vi "Function_Generator2.vi"() -> ()   [LabVIEW 2013]
uses:
  <vilib>/express/express analysis/Spectral/Block/exnSpectralBlock spectral measurements peak poly.vi
  <vilib>/express/express analysis/Spectral/Block/exnSpectralBlock spectral measurements peak DDT.vi
  <vilib>/express/express analysis/Spectral/XNode/ExpressSpectralMeasurementsBlockNode.xnode
panel:
  out ".not. x?":bool
  in  "File save selector":T1(radio)
  out "Recorded time":dbl
  in  "Record & Stop Button":bool
  in  "Radio Buttons":T1(radio)
  in  "Jpg imgae button":bool
  in  "Tab Control":enum32{"Waveform", "FFT"}(tab)
  out "Waveform Graph 2":dynamicdata(graph) caption="Waveform Graph"
  out "FFT":dynamicdata(graph)
  in  "Noise on/off":bool
  in  "ms/Div":i32(knob) scale=0.0..4.0 scale format="%.0g"
  in  "Volt/Div":dbl(knob) scale=0.0..4.0 scale format="%_2g"
  in  "Offset":i32(slide) scale=-5.0..5.0
  in  "Frequency":dbl(knob) scale=10.0..20.0 scale format="%#_2p"
  in  "Freq mutiplier":dbl(slide) caption="Multiplier" scale=2.0..1000.0
  in  "Trigger":bool
  out "DC":bool
  out "Square":bool
  out "Sawtooth":bool
  out "Traingle":bool
  out "Sine":bool
  out "Frequency":dbl format="%#_3pHz"
  out "Peak to Peak Amplitude":dbl format="%#_3gV"
  in  "Noise":i32(knob) scale=0.0..2.0
  in  "Phase":dbl(knob) scale=0.0..360.0 scale format="%.0p"
  in  "Signal type":i32(knob) step=1 scale=0.0..4.0
  in  "Amplitude":dbl(knob) scale=0.0..10.0
  in  "stop":bool
  in  "Duty Cycle (%)":dbl(knob)=50.0 scale=0.0..100.0
  in  "Standered deviation":dbl(slide) scale=-1.0..1.0 scale format="%#_1g"
  in  "Noise Amplitude":dbl(slide) scale=0.0..5.0
  in  "FFT save button":bool
  in  "Trail probability":dbl(slide) scale=0.0..1.0 scale format="%#.1g"
  # "Function Generator / Oscilloscope"
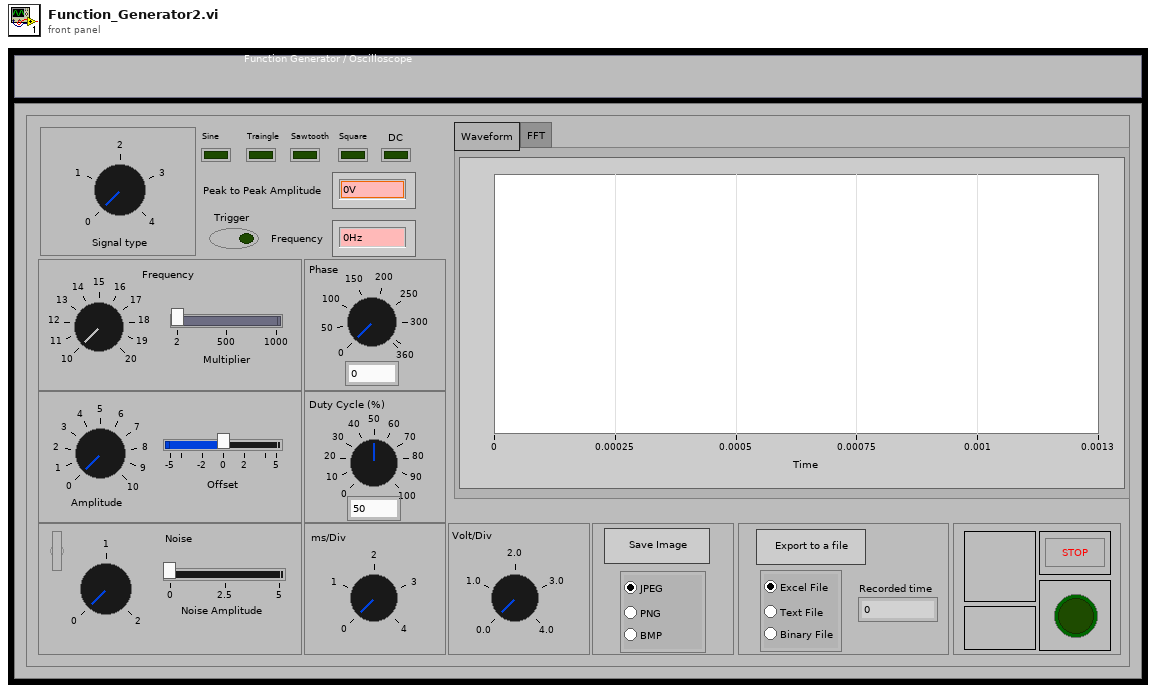
[diagram p1: front panel]
types:
  T1 = enum32{"Radio Selection 1", "Radio Selection 2", "Radio Selection 3"}
  T2 = cluster{"averaging mode":u16, "weighting mode":u16, "number of averages":u32}
  T3 = cluster{"dB On (F)":bool, "unwrap phase (F)":bool, "convert to degree (F)":bool}
  T4 = typedef "imagedata.ctl" = cluster{"image type":i32, "image depth":i32, "image":u8[], "mask":u8[], "colors":u32[], "Rectangle":cluster{"left":i16, "top":i16, "right":i16, "bottom":i16}}
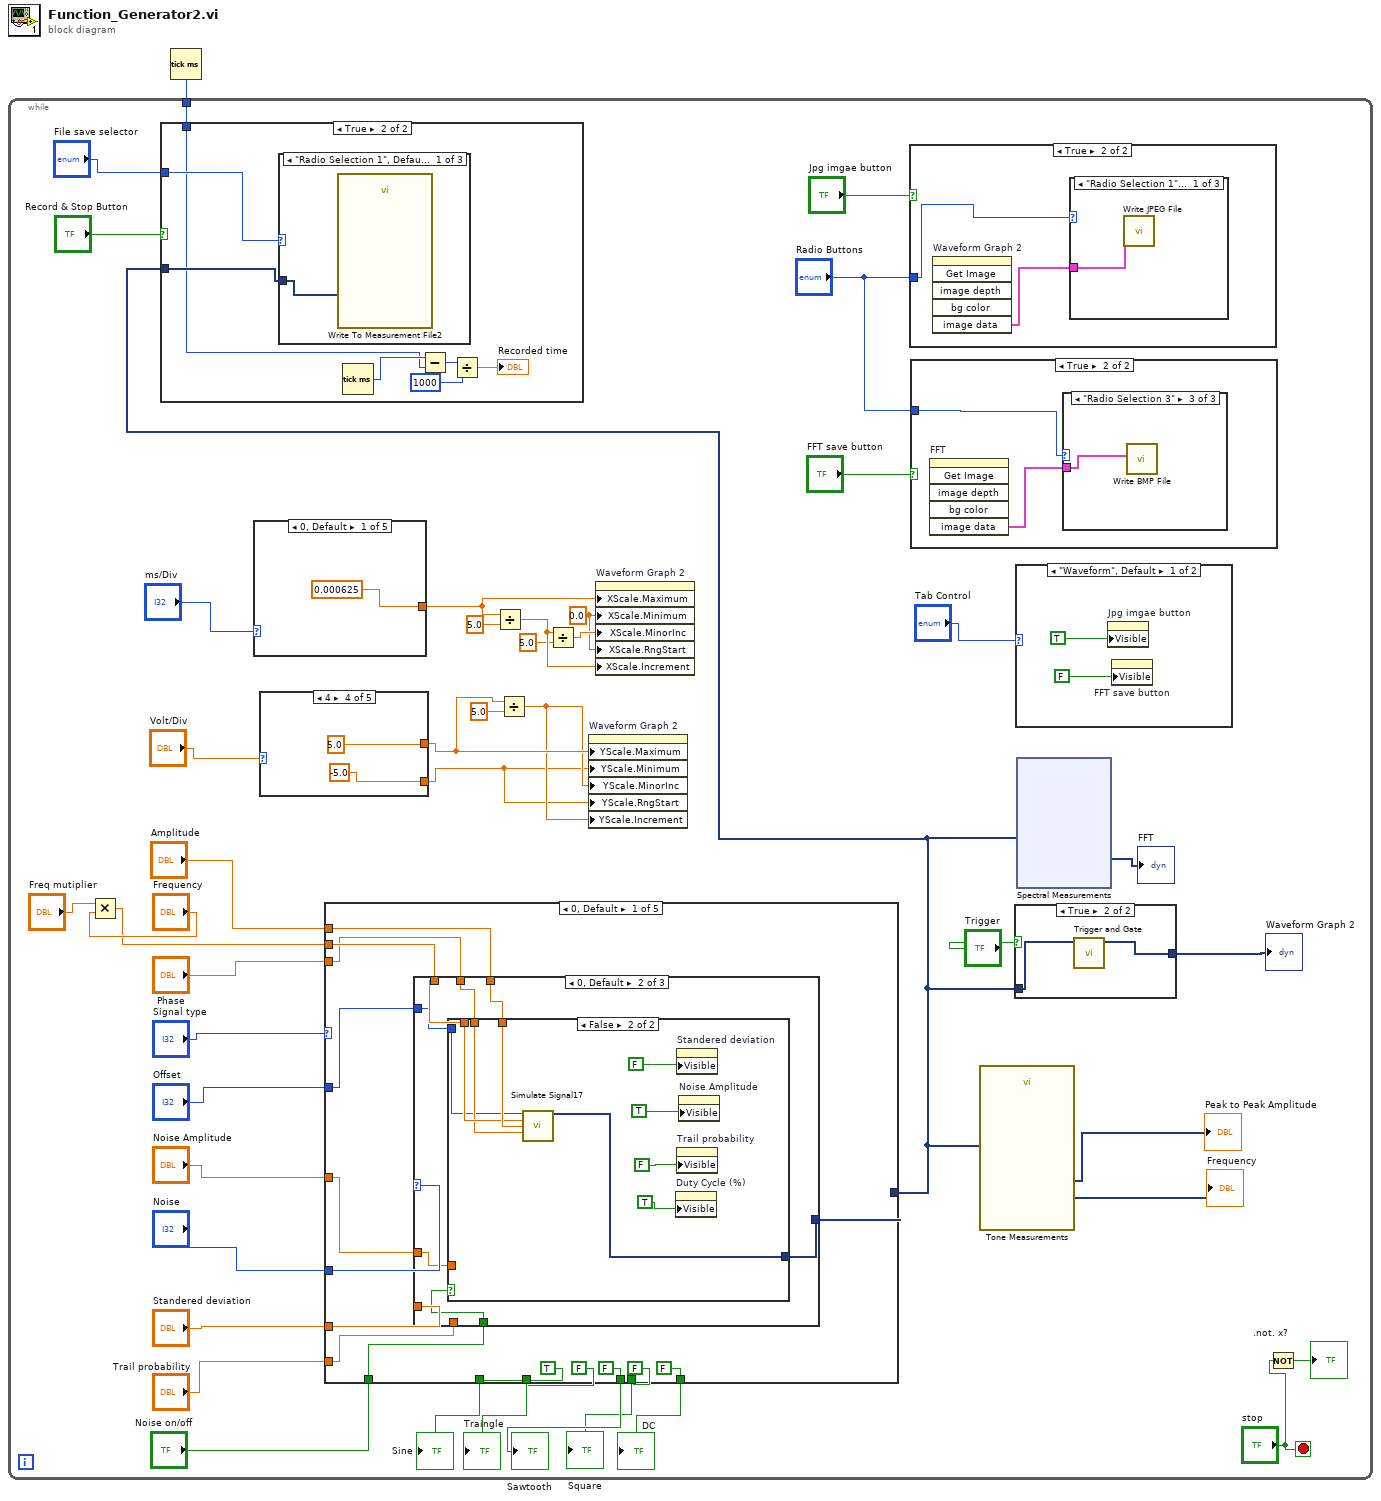
[diagram p0: block diagram]
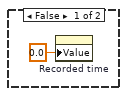
[diagram p2: hidden frame]
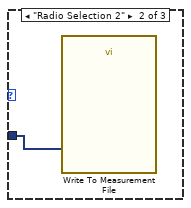
[diagram p3: hidden frame]
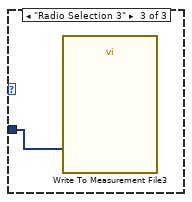
[diagram p4: hidden frame]
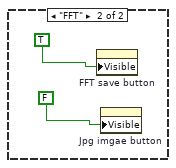
[diagram p5: hidden frame]
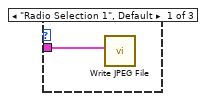
[diagram p7: hidden frame]
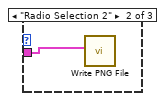
[diagram p8: hidden frame]
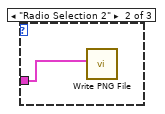
[diagram p10: hidden frame]
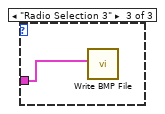
[diagram p11: hidden frame]
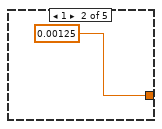
[diagram p12: hidden frame]
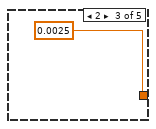
[diagram p13: hidden frame]
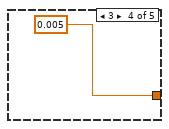
[diagram p14: hidden frame]
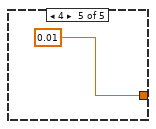
[diagram p15: hidden frame]
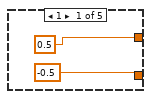
[diagram p16: hidden frame]
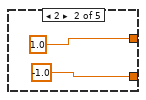
[diagram p17: hidden frame]
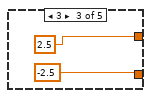
[diagram p18: hidden frame]
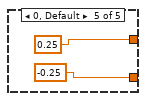
[diagram p19: hidden frame]
diagram:
  n1 = Tick Count (ms)() -> (millisecond timer value=w1:u32)
  n2 = while {
    tunnel: w1 -> [w6]
    stop <- "stop" stop-if-true
    w14 = 0.0 ("X Scale.Range:Minimum")
    n3 = Multiply(x="Freq mutiplier", y="Frequency") -> (x*y=w27:dbl)
    n4 = case shown="0, Default" "ms/Div" {
      tunnel: [0.000625 0.00125 0.0025 0.005 0.01] -> w19
      frame 0, Default {
      }
      frame 1 {
      }
      frame 2 {
      }
      frame 3 {
      }
      frame 4 {
      }
    }
    n5 = case shown="4" "Volt/Div" {
      tunnel: [0.5 1.0 2.5 5.0 0.25] -> w23
      tunnel: [-0.5 -1.0 -2.5 -5.0 -0.25] -> w21
      frame 1 {
      }
      frame 2 {
      }
      frame 3 {
      }
      frame 4 {
      }
      frame 0, Default {
      }
    }
    n6 = case shown="0, Default" "Signal type" {
      tunnel: "Amplitude" -> [w113 w204 w298 w389 _]
      tunnel: w27 -> [w112 w203 w297 w388 _]
      tunnel: "Phase" -> [w111 w202 w296 w387 _]
      tunnel: "Offset" -> [w110 w199 w295 w386 w488]
      tunnel: "Noise Amplitude" -> [w108 w205 w294 w385 w487]
      tunnel: "Noise" -> [w105 w206 w299 w390 w489]
      tunnel: "Standered deviation" -> [w109 w200 w292 w383 w485]
      tunnel: "Trail probability" -> [w107 w198 w291 w382 w484]
      tunnel: [w106 w201 w293 w384 w486] -> w7
      tunnel: [TRUE FALSE FALSE FALSE FALSE] -> w36
      tunnel: [FALSE TRUE FALSE FALSE FALSE] -> w35
      tunnel: [FALSE FALSE TRUE FALSE FALSE] -> w34
      tunnel: [FALSE FALSE FALSE TRUE FALSE] -> w33
      tunnel: [FALSE FALSE FALSE FALSE TRUE] -> w32
      tunnel: "Noise on/off" -> [w99 w192 w285 w375 w478]
      frame 0, Default {
        n7 = case shown="0, Default" w105 {
          tunnel: w113 -> [w120 w146 w172]
          tunnel: w112 -> [w118 w145 w171]
          tunnel: w111 -> [w119 w144 w170]
          tunnel: w110 -> [w115 w143 w169]
          tunnel: w109 -> [_ _ w168]
          tunnel: w108 -> [_ w142 _]
          tunnel: w107 -> [w117 _ _]
          tunnel: [w116 w141 w167] -> w106
          tunnel: w99 -> [w114 w140 w166]
          frame 2 {
            n8 = case shown="False" w114 {
              tunnel: w120 -> [w130 w139]
              tunnel: w119 -> [w129 w138]
              tunnel: w118 -> [w128 w137]
              tunnel: w117 -> [w127 _]
              tunnel: [w123 w133] -> w116
              tunnel: w115 -> [w121 w131]
              frame True {
                n9 = call "Simulate Signal3"("Offset"=w121, "Frequency"=w128, "Amplitude"=w130, "Phase"=w129, "Trial probability"=w127) -> ("Sine with Binomial Noise"=w123:dynamicdata)  [unwired: 9 in, 1 out]
                n10 = property on="Duty Cycle (%)" class="Knob (strict)"("Visible"=TRUE) -> ()  [unwired: 2 in, 2 out]
                n11 = property on="Noise Amplitude" class="Slide (strict)"("Visible"=FALSE) -> ()  [unwired: 2 in, 2 out]
                n12 = property on="Trail probability" class="Slide (strict)"("Visible"=TRUE) -> ()  [unwired: 2 in, 2 out]
                n13 = property on="Standered deviation" class="Slide (strict)"("Visible"=FALSE) -> ()  [unwired: 2 in, 2 out]
              }
              frame False {
                n14 = call "Simulate Signal18"("Offset"=w131, "Frequency"=w137, "Amplitude"=w139, "Phase"=w138) -> ("Sine"=w133:dynamicdata)  [unwired: 10 in, 1 out]
                n15 = property on="Duty Cycle (%)" class="Knob (strict)"("Visible"=TRUE) -> ()  [unwired: 2 in, 2 out]
                n16 = property on="Noise Amplitude" class="Slide (strict)"("Visible"=FALSE) -> ()  [unwired: 2 in, 2 out]
                n17 = property on="Trail probability" class="Slide (strict)"("Visible"=TRUE) -> ()  [unwired: 2 in, 2 out]
                n18 = property on="Standered deviation" class="Slide (strict)"("Visible"=FALSE) -> ()  [unwired: 2 in, 2 out]
              }
            }
          }
          frame 0, Default {
            n19 = case shown="False" w140 {
              tunnel: w146 -> [w156 w165]
              tunnel: w145 -> [w155 w164]
              tunnel: w144 -> [w154 w163]
              tunnel: w143 -> [w153 w162]
              tunnel: w142 -> [w152 _]
              tunnel: [w148 w158] -> w141
              frame True {
                n20 = call "Simulate Signal"("Offset"=w153, "Frequency"=w155, "Amplitude"=w156, "Phase"=w154, "Noise amplitude"=w152) -> ("Sine with Uniform Noise"=w148:dynamicdata)  [unwired: 9 in, 1 out]
                n21 = property on="Duty Cycle (%)" class="Knob (strict)"("Visible"=TRUE) -> ()  [unwired: 2 in, 2 out]
                n22 = property on="Standered deviation" class="Slide (strict)"("Visible"=FALSE) -> ()  [unwired: 2 in, 2 out]
                n23 = property on="Trail probability" class="Slide (strict)"("Visible"=FALSE) -> ()  [unwired: 2 in, 2 out]
                n24 = property on="Noise Amplitude" class="Slide (strict)"("Visible"=TRUE) -> ()  [unwired: 2 in, 2 out]
              }
              frame False {
                n25 = call "Simulate Signal17"("Offset"=w162, "Frequency"=w164, "Amplitude"=w165, "Phase"=w163) -> ("Sine"=w158:dynamicdata)  [unwired: 10 in, 1 out]
                n26 = property on="Duty Cycle (%)" class="Knob (strict)"("Visible"=TRUE) -> ()  [unwired: 2 in, 2 out]
                n27 = property on="Standered deviation" class="Slide (strict)"("Visible"=FALSE) -> ()  [unwired: 2 in, 2 out]
                n28 = property on="Trail probability" class="Slide (strict)"("Visible"=FALSE) -> ()  [unwired: 2 in, 2 out]
                n29 = property on="Noise Amplitude" class="Slide (strict)"("Visible"=TRUE) -> ()  [unwired: 2 in, 2 out]
              }
            }
          }
          frame 1 {
            n30 = case shown="True" w166 {
              tunnel: w172 -> [w182 w191]
              tunnel: w171 -> [w181 w190]
              tunnel: w170 -> [w180 w189]
              tunnel: w169 -> [w179 w188]
              tunnel: w168 -> [w178 _]
              tunnel: [w174 w184] -> w167
              frame True {
                n31 = call "Simulate Signal2"("Offset"=w179, "Frequency"=w181, "Amplitude"=w182, "Phase"=w180, "Standard deviation"=w178) -> ("Sine with Gaussian Noise"=w174:dynamicdata)  [unwired: 9 in, 1 out]
                n32 = property on="Noise Amplitude" class="Slide (strict)"("Visible"=FALSE) -> ()  [unwired: 2 in, 2 out]
                n33 = property on="Standered deviation" class="Slide (strict)"("Visible"=TRUE) -> ()  [unwired: 2 in, 2 out]
                n34 = property on="Trail probability" class="Slide (strict)"("Visible"=FALSE) -> ()  [unwired: 2 in, 2 out]
                n35 = property on="Duty Cycle (%)" class="Knob (strict)"("Visible"=TRUE) -> ()  [unwired: 2 in, 2 out]
              }
              frame False {
                n36 = call "Simulate Signal16"("Offset"=w188, "Frequency"=w190, "Amplitude"=w191, "Phase"=w189) -> ("Sine"=w184:dynamicdata)  [unwired: 10 in, 1 out]
                n37 = property on="Noise Amplitude" class="Slide (strict)"("Visible"=FALSE) -> ()  [unwired: 2 in, 2 out]
                n38 = property on="Standered deviation" class="Slide (strict)"("Visible"=TRUE) -> ()  [unwired: 2 in, 2 out]
                n39 = property on="Trail probability" class="Slide (strict)"("Visible"=FALSE) -> ()  [unwired: 2 in, 2 out]
                n40 = property on="Duty Cycle (%)" class="Knob (strict)"("Visible"=TRUE) -> ()  [unwired: 2 in, 2 out]
              }
            }
          }
        }
      }
      frame 1 {
        n41 = case shown="1" w206 {
          tunnel: w205 -> [w213 _ w261]
          tunnel: w204 -> [w212 w238 w264]
          tunnel: w203 -> [w211 w237 w263]
          tunnel: w202 -> [w210 w236 w262]
          tunnel: [w209 w234 w260] -> w201
          tunnel: w200 -> [_ w239 _]
          tunnel: w199 -> [w208 w235 _]
          tunnel: w198 -> [_ _ w265]
          tunnel: w192 -> [w207 w233 w259]
          frame 0, Default {
            n42 = case shown="False" w207 {
              tunnel: w213 -> [w223 _]
              tunnel: w212 -> [w222 w232]
              tunnel: w211 -> [w221 w231]
              tunnel: w210 -> [w220 w230]
              tunnel: [w219 w229] -> w209
              tunnel: w208 -> [w215 w225]
              frame True {
                n43 = call "Simulate Signal4"("Offset"=w215, "Frequency"=w221, "Amplitude"=w222, "Phase"=w220, "Noise amplitude"=w223) -> ("Triangle with Uniform Noise"=w219:dynamicdata)  [unwired: 9 in, 1 out]
                n44 = property on="Standered deviation" class="Slide (strict)"("Visible"=FALSE) -> ()  [unwired: 2 in, 2 out]
                n45 = property on="Noise Amplitude" class="Slide (strict)"("Visible"=TRUE) -> ()  [unwired: 2 in, 2 out]
                n46 = property on="Trail probability" class="Slide (strict)"("Visible"=FALSE) -> ()  [unwired: 2 in, 2 out]
                n47 = property on="Duty Cycle (%)" class="Knob (strict)"("Visible"=TRUE) -> ()  [unwired: 2 in, 2 out]
              }
              frame False {
                n48 = call "Simulate Signal21"("Offset"=w225, "Frequency"=w231, "Amplitude"=w232, "Phase"=w230) -> ("Triangle"=w229:dynamicdata)  [unwired: 10 in, 1 out]
                n49 = property on="Standered deviation" class="Slide (strict)"("Visible"=FALSE) -> ()  [unwired: 2 in, 2 out]
                n50 = property on="Noise Amplitude" class="Slide (strict)"("Visible"=TRUE) -> ()  [unwired: 2 in, 2 out]
                n51 = property on="Trail probability" class="Slide (strict)"("Visible"=FALSE) -> ()  [unwired: 2 in, 2 out]
                n52 = property on="Duty Cycle (%)" class="Knob (strict)"("Visible"=TRUE) -> ()  [unwired: 2 in, 2 out]
              }
            }
          }
          frame 1 {
            n53 = case shown="True" w233 {
              tunnel: w239 -> [w249 _]
              tunnel: w238 -> [w248 w258]
              tunnel: w237 -> [w247 w257]
              tunnel: w236 -> [w246 w256]
              tunnel: w235 -> [w245 w255]
              tunnel: [w244 w254] -> w234
              frame True {
                n54 = call "Simulate Signal5"("Offset"=w245, "Frequency"=w247, "Amplitude"=w248, "Phase"=w246, "Standard deviation"=w249) -> ("Triangle with Gaussian Noise"=w244:dynamicdata)  [unwired: 9 in, 1 out]
                n55 = property on="Noise Amplitude" class="Slide (strict)"("Visible"=FALSE) -> ()  [unwired: 2 in, 2 out]
                n56 = property on="Standered deviation" class="Slide (strict)"("Visible"=TRUE) -> ()  [unwired: 2 in, 2 out]
                n57 = property on="Trail probability" class="Slide (strict)"("Visible"=FALSE) -> ()  [unwired: 2 in, 2 out]
                n58 = property on="Duty Cycle (%)" class="Knob (strict)"("Visible"=TRUE) -> ()  [unwired: 2 in, 2 out]
              }
              frame False {
                n59 = call "Simulate Signal19"("Offset"=w255, "Frequency"=w257, "Amplitude"=w258, "Phase"=w256) -> ("Triangle"=w254:dynamicdata)  [unwired: 10 in, 1 out]
                n60 = property on="Noise Amplitude" class="Slide (strict)"("Visible"=FALSE) -> ()  [unwired: 2 in, 2 out]
                n61 = property on="Standered deviation" class="Slide (strict)"("Visible"=TRUE) -> ()  [unwired: 2 in, 2 out]
                n62 = property on="Trail probability" class="Slide (strict)"("Visible"=FALSE) -> ()  [unwired: 2 in, 2 out]
                n63 = property on="Duty Cycle (%)" class="Knob (strict)"("Visible"=TRUE) -> ()  [unwired: 2 in, 2 out]
              }
            }
          }
          frame 2 {
            n64 = case shown="False" w259 {
              tunnel: w265 -> [w275 _]
              tunnel: w264 -> [w274 w284]
              tunnel: w263 -> [w273 w283]
              tunnel: w262 -> [w272 w282]
              tunnel: w261 -> [w271 w281]
              tunnel: [w270 w280] -> w260
              frame True {
                n65 = call "Simulate Signal6"("Offset"=w271, "Frequency"=w273, "Amplitude"=w274, "Phase"=w272, "Trial probability"=w275) -> ("Triangle with Binomial Noise"=w270:dynamicdata)  [unwired: 9 in, 1 out]
                n66 = property on="Duty Cycle (%)" class="Knob (strict)"("Visible"=TRUE) -> ()  [unwired: 2 in, 2 out]
                n67 = property on="Noise Amplitude" class="Slide (strict)"("Visible"=FALSE) -> ()  [unwired: 2 in, 2 out]
                n68 = property on="Standered deviation" class="Slide (strict)"("Visible"=FALSE) -> ()  [unwired: 2 in, 2 out]
                n69 = property on="Trail probability" class="Slide (strict)"("Visible"=TRUE) -> ()  [unwired: 2 in, 2 out]
              }
              frame False {
                n70 = call "Simulate Signal20"("Offset"=w281, "Frequency"=w283, "Amplitude"=w284, "Phase"=w282) -> ("Triangle"=w280:dynamicdata)  [unwired: 10 in, 1 out]
                n71 = property on="Duty Cycle (%)" class="Knob (strict)"("Visible"=TRUE) -> ()  [unwired: 2 in, 2 out]
                n72 = property on="Noise Amplitude" class="Slide (strict)"("Visible"=FALSE) -> ()  [unwired: 2 in, 2 out]
                n73 = property on="Standered deviation" class="Slide (strict)"("Visible"=FALSE) -> ()  [unwired: 2 in, 2 out]
                n74 = property on="Trail probability" class="Slide (strict)"("Visible"=TRUE) -> ()  [unwired: 2 in, 2 out]
              }
            }
          }
        }
      }
      frame 2 {
        n75 = case shown="1" w299 {
          tunnel: w298 -> [w306 w332 w357]
          tunnel: w297 -> [w305 w331 w356]
          tunnel: w296 -> [w304 w330 _]
          tunnel: w295 -> [w303 w329 w355]
          tunnel: w294 -> [w302 _ _]
          tunnel: [w301 w327 w353] -> w293
          tunnel: w292 -> [_ w328 _]
          tunnel: w291 -> [_ _ w354]
          tunnel: w285 -> [w300 w326 w352]
          frame 0, Default {
            n76 = case shown="False" w300 {
              tunnel: w306 -> [w316 w325]
              tunnel: w305 -> [w315 w324]
              tunnel: w304 -> [w314 w323]
              tunnel: w303 -> [w313 w322]
              tunnel: w302 -> [w312 _]
              tunnel: [w311 w321] -> w301
              frame True {
                n77 = call "Simulate Signal7"("Offset"=w313, "Frequency"=w315, "Amplitude"=w316, "Phase"=w314, "Noise amplitude"=w312) -> ("Sawtooth with Uniform Noise"=w311:dynamicdata)  [unwired: 9 in, 1 out]
                n78 = property on="Standered deviation" class="Slide (strict)"("Visible"=FALSE) -> ()  [unwired: 2 in, 2 out]
                n79 = property on="Trail probability" class="Slide (strict)"("Visible"=FALSE) -> ()  [unwired: 2 in, 2 out]
                n80 = property on="Duty Cycle (%)" class="Knob (strict)"("Visible"=TRUE) -> ()  [unwired: 2 in, 2 out]
                n81 = property on="Noise Amplitude" class="Slide (strict)"("Visible"=TRUE) -> ()  [unwired: 2 in, 2 out]
              }
              frame False {
                n82 = call "Simulate Signal22"("Offset"=w322, "Frequency"=w324, "Amplitude"=w325, "Phase"=w323) -> ("Sawtooth"=w321:dynamicdata)  [unwired: 10 in, 1 out]
                n83 = property on="Standered deviation" class="Slide (strict)"("Visible"=FALSE) -> ()  [unwired: 2 in, 2 out]
                n84 = property on="Trail probability" class="Slide (strict)"("Visible"=FALSE) -> ()  [unwired: 2 in, 2 out]
                n85 = property on="Duty Cycle (%)" class="Knob (strict)"("Visible"=TRUE) -> ()  [unwired: 2 in, 2 out]
                n86 = property on="Noise Amplitude" class="Slide (strict)"("Visible"=TRUE) -> ()  [unwired: 2 in, 2 out]
              }
            }
          }
          frame 1 {
            n87 = case shown="True" w326 {
              tunnel: w332 -> [w342 w351]
              tunnel: w331 -> [w341 w350]
              tunnel: w330 -> [w340 w349]
              tunnel: w329 -> [w339 w348]
              tunnel: w328 -> [w338 _]
              tunnel: [w337 w347] -> w327
              frame True {
                n88 = call "Simulate Signal8"("Offset"=w339, "Frequency"=w341, "Amplitude"=w342, "Phase"=w340, "Standard deviation"=w338) -> ("Sawtooth with Gaussian Noise"=w337:dynamicdata)  [unwired: 9 in, 1 out]
                n89 = property on="Noise Amplitude" class="Slide (strict)"("Visible"=FALSE) -> ()  [unwired: 2 in, 2 out]
                n90 = property on="Trail probability" class="Slide (strict)"("Visible"=FALSE) -> ()  [unwired: 2 in, 2 out]
                n91 = property on="Duty Cycle (%)" class="Knob (strict)"("Visible"=TRUE) -> ()  [unwired: 2 in, 2 out]
                n92 = property on="Standered deviation" class="Slide (strict)"("Visible"=TRUE) -> ()  [unwired: 2 in, 2 out]
              }
              frame False {
                n93 = call "Simulate Signal23"("Offset"=w348, "Frequency"=w350, "Amplitude"=w351, "Phase"=w349) -> ("Sawtooth"=w347:dynamicdata)  [unwired: 10 in, 1 out]
                n94 = property on="Noise Amplitude" class="Slide (strict)"("Visible"=FALSE) -> ()  [unwired: 2 in, 2 out]
                n95 = property on="Trail probability" class="Slide (strict)"("Visible"=FALSE) -> ()  [unwired: 2 in, 2 out]
                n96 = property on="Duty Cycle (%)" class="Knob (strict)"("Visible"=TRUE) -> ()  [unwired: 2 in, 2 out]
                n97 = property on="Standered deviation" class="Slide (strict)"("Visible"=TRUE) -> ()  [unwired: 2 in, 2 out]
              }
            }
          }
          frame 2 {
            n98 = case shown="True" w352 {
              tunnel: w357 -> [w366 w374]
              tunnel: w356 -> [w365 w373]
              tunnel: w355 -> [w364 w372]
              tunnel: w354 -> [w363 _]
              tunnel: [w362 w371] -> w353
              frame True {
                n99 = call "Simulate Signal9"("Offset"=w364, "Frequency"=w365, "Amplitude"=w366, "Trial probability"=w363) -> ("Sawtooth with Binomial Noise"=w362:dynamicdata)  [unwired: 10 in, 1 out]
                n100 = property on="Duty Cycle (%)" class="Knob (strict)"("Visible"=TRUE) -> ()  [unwired: 2 in, 2 out]
                n101 = property on="Noise Amplitude" class="Slide (strict)"("Visible"=FALSE) -> ()  [unwired: 2 in, 2 out]
                n102 = property on="Standered deviation" class="Slide (strict)"("Visible"=FALSE) -> ()  [unwired: 2 in, 2 out]
                n103 = property on="Trail probability" class="Slide (strict)"("Visible"=TRUE) -> ()  [unwired: 2 in, 2 out]
              }
              frame False {
                n104 = call "Simulate Signal24"("Offset"=w372, "Frequency"=w373, "Amplitude"=w374) -> ("Sawtooth"=w371:dynamicdata)  [unwired: 11 in, 1 out]
                n105 = property on="Duty Cycle (%)" class="Knob (strict)"("Visible"=TRUE) -> ()  [unwired: 2 in, 2 out]
                n106 = property on="Noise Amplitude" class="Slide (strict)"("Visible"=FALSE) -> ()  [unwired: 2 in, 2 out]
                n107 = property on="Standered deviation" class="Slide (strict)"("Visible"=FALSE) -> ()  [unwired: 2 in, 2 out]
                n108 = property on="Trail probability" class="Slide (strict)"("Visible"=TRUE) -> ()  [unwired: 2 in, 2 out]
              }
            }
          }
        }
      }
      frame 3 {
        n109 = case shown="1" w390 {
          tunnel: w389 -> [w398 w427 w456]
          tunnel: w388 -> [w397 w426 w455]
          tunnel: w387 -> [w396 w424 w453]
          tunnel: w386 -> [w395 w425 w454]
          tunnel: w385 -> [w394 _ _]
          tunnel: [w393 w422 w451] -> w384
          tunnel: w383 -> [_ w423 _]
          tunnel: w382 -> [_ _ w452]
          tunnel: "Duty Cycle (%)" -> [w392 w421 w450]
          tunnel: w375 -> [w391 w420 w449]
          frame 0, Default {
            n110 = case shown="False" w391 {
              tunnel: w398 -> [w409 w419]
              tunnel: w397 -> [w408 w418]
              tunnel: w396 -> [w407 w417]
              tunnel: w395 -> [w406 w416]
              tunnel: w394 -> [w405 _]
              tunnel: [w404 w415] -> w393
              tunnel: w392 -> [w400 w411]
              frame True {
                n111 = call "Simulate Signal10"("Offset"=w406, "Duty Cycle (%)"=w400, "Frequency"=w408, "Amplitude"=w409, "Phase"=w407, "Noise amplitude"=w405) -> ("Square with Uniform Noise"=w404:dynamicdata)  [unwired: 8 in, 1 out]
                n112 = property on="Duty Cycle (%)" class="Knob (strict)"("Visible"=TRUE) -> ()  [unwired: 2 in, 2 out]
                n113 = property on="Standered deviation" class="Slide (strict)"("Visible"=FALSE) -> ()  [unwired: 2 in, 2 out]
                n114 = property on="Trail probability" class="Slide (strict)"("Visible"=FALSE) -> ()  [unwired: 2 in, 2 out]
                n115 = property on="Noise Amplitude" class="Slide (strict)"("Visible"=TRUE) -> ()  [unwired: 2 in, 2 out]
              }
              frame False {
                n116 = call "Simulate Signal27"("Offset"=w416, "Duty Cycle (%)"=w411, "Frequency"=w418, "Amplitude"=w419, "Phase"=w417) -> ("Square"=w415:dynamicdata)  [unwired: 9 in, 1 out]
                n117 = property on="Duty Cycle (%)" class="Knob (strict)"("Visible"=TRUE) -> ()  [unwired: 2 in, 2 out]
                n118 = property on="Standered deviation" class="Slide (strict)"("Visible"=FALSE) -> ()  [unwired: 2 in, 2 out]
                n119 = property on="Trail probability" class="Slide (strict)"("Visible"=FALSE) -> ()  [unwired: 2 in, 2 out]
                n120 = property on="Noise Amplitude" class="Slide (strict)"("Visible"=TRUE) -> ()  [unwired: 2 in, 2 out]
              }
            }
          }
          frame 1 {
            n121 = case shown="False" w420 {
              tunnel: w427 -> [w435 w445]
              tunnel: w426 -> [w434 w444]
              tunnel: w425 -> [w433 w443]
              tunnel: w424 -> [w432 w442]
              tunnel: w423 -> [w431 _]
              tunnel: [w430 w441] -> w422
              tunnel: w421 -> [w429 w440]
              frame True {
                n122 = call "Simulate Signal11"("Offset"=w433, "Duty Cycle (%)"=w429, "Frequency"=w434, "Amplitude"=w435, "Phase"=w432, "Standard deviation"=w431) -> ("Square with Gaussian Noise"=w430:dynamicdata)  [unwired: 8 in, 1 out]
                n123 = property on="Duty Cycle (%)" class="Knob (strict)"("Visible"=TRUE) -> ()  [unwired: 2 in, 2 out]
                n124 = property on="Noise Amplitude" class="Slide (strict)"("Visible"=FALSE) -> ()  [unwired: 2 in, 2 out]
                n125 = property on="Trail probability" class="Slide (strict)"("Visible"=FALSE) -> ()  [unwired: 2 in, 2 out]
                n126 = property on="Standered deviation" class="Slide (strict)"("Visible"=TRUE) -> ()  [unwired: 2 in, 2 out]
              }
              frame False {
                n127 = call "Simulate Signal25"("Offset"=w443, "Duty Cycle (%)"=w440, "Frequency"=w444, "Amplitude"=w445, "Phase"=w442) -> ("Square"=w441:dynamicdata)  [unwired: 9 in, 1 out]
                n128 = property on="Duty Cycle (%)" class="Knob (strict)"("Visible"=TRUE) -> ()  [unwired: 2 in, 2 out]
                n129 = property on="Noise Amplitude" class="Slide (strict)"("Visible"=FALSE) -> ()  [unwired: 2 in, 2 out]
                n130 = property on="Trail probability" class="Slide (strict)"("Visible"=FALSE) -> ()  [unwired: 2 in, 2 out]
                n131 = property on="Standered deviation" class="Slide (strict)"("Visible"=TRUE) -> ()  [unwired: 2 in, 2 out]
              }
            }
          }
          frame 2 {
            n132 = case shown="False" w449 {
              tunnel: w456 -> [w467 w477]
              tunnel: w455 -> [w466 w476]
              tunnel: w454 -> [w465 w475]
              tunnel: w453 -> [w464 w474]
              tunnel: w452 -> [w463 _]
              tunnel: [w459 w470] -> w451
              tunnel: w450 -> [w458 w469]
              frame True {
                n133 = call "Simulate Signal12"("Offset"=w465, "Duty Cycle (%)"=w458, "Frequency"=w466, "Amplitude"=w467, "Phase"=w464, "Trial probability"=w463) -> ("Square with Binomial Noise"=w459:dynamicdata)  [unwired: 8 in, 1 out]
                n134 = property on="Noise Amplitude" class="Slide (strict)"("Visible"=FALSE) -> ()  [unwired: 2 in, 2 out]
                n135 = property on="Standered deviation" class="Slide (strict)"("Visible"=FALSE) -> ()  [unwired: 2 in, 2 out]
                n136 = property on="Trail probability" class="Slide (strict)"("Visible"=TRUE) -> ()  [unwired: 2 in, 2 out]
                n137 = property on="Duty Cycle (%)" class="Knob (strict)"("Visible"=TRUE) -> ()  [unwired: 2 in, 2 out]
              }
              frame False {
                n138 = call "Simulate Signal26"("Offset"=w475, "Duty Cycle (%)"=w469, "Frequency"=w476, "Amplitude"=w477, "Phase"=w474) -> ("Square"=w470:dynamicdata)  [unwired: 9 in, 1 out]
                n139 = property on="Noise Amplitude" class="Slide (strict)"("Visible"=FALSE) -> ()  [unwired: 2 in, 2 out]
                n140 = property on="Standered deviation" class="Slide (strict)"("Visible"=FALSE) -> ()  [unwired: 2 in, 2 out]
                n141 = property on="Trail probability" class="Slide (strict)"("Visible"=TRUE) -> ()  [unwired: 2 in, 2 out]
                n142 = property on="Duty Cycle (%)" class="Knob (strict)"("Visible"=TRUE) -> ()  [unwired: 2 in, 2 out]
              }
            }
          }
        }
      }
      frame 4 {
        n143 = case shown="0, Default" w489 {
          tunnel: w488 -> [w493 w510 w527]
          tunnel: w487 -> [w492 _ _]
          tunnel: [w491 w508 w525] -> w486
          tunnel: w485 -> [_ w509 _]
          tunnel: w484 -> [_ _ w526]
          tunnel: w478 -> [w490 w507 w524]
          frame 0, Default {
            n144 = case shown="False" w490 {
              tunnel: w493 -> [w500 w506]
              tunnel: w492 -> [w499 _]
              tunnel: [w498 w505] -> w491
              frame True {
                n145 = call "Simulate Signal13"("Offset"=w500, "Noise amplitude"=w499) -> ("DC with Uniform Noise"=w498:dynamicdata)  [unwired: 12 in, 1 out]
                n146 = property on="Standered deviation" class="Slide (strict)"("Visible"=FALSE) -> ()  [unwired: 2 in, 2 out]
                n147 = property on="Noise Amplitude" class="Slide (strict)"("Visible"=TRUE) -> ()  [unwired: 2 in, 2 out]
                n148 = property on="Trail probability" class="Slide (strict)"("Visible"=FALSE) -> ()  [unwired: 2 in, 2 out]
                n149 = property on="Duty Cycle (%)" class="Knob (strict)"("Visible"=TRUE) -> ()  [unwired: 2 in, 2 out]
              }
              frame False {
                n150 = call "Simulate Signal28"("Offset"=w506) -> ("DC"=w505:dynamicdata)  [unwired: 13 in, 1 out]
                n151 = property on="Standered deviation" class="Slide (strict)"("Visible"=FALSE) -> ()  [unwired: 2 in, 2 out]
                n152 = property on="Noise Amplitude" class="Slide (strict)"("Visible"=TRUE) -> ()  [unwired: 2 in, 2 out]
                n153 = property on="Trail probability" class="Slide (strict)"("Visible"=FALSE) -> ()  [unwired: 2 in, 2 out]
                n154 = property on="Duty Cycle (%)" class="Knob (strict)"("Visible"=TRUE) -> ()  [unwired: 2 in, 2 out]
              }
            }
          }
          frame 1 {
            n155 = case shown="False" w507 {
              tunnel: w510 -> [w517 w523]
              tunnel: w509 -> [w516 _]
              tunnel: [w515 w522] -> w508
              frame True {
                n156 = call "Simulate Signal14"("Offset"=w517, "Standard deviation"=w516) -> ("DC with Gaussian Noise"=w515:dynamicdata)  [unwired: 12 in, 1 out]
                n157 = property on="Noise Amplitude" class="Slide (strict)"("Visible"=FALSE) -> ()  [unwired: 2 in, 2 out]
                n158 = property on="Trail probability" class="Slide (strict)"("Visible"=FALSE) -> ()  [unwired: 2 in, 2 out]
                n159 = property on="Duty Cycle (%)" class="Knob (strict)"("Visible"=TRUE) -> ()  [unwired: 2 in, 2 out]
                n160 = property on="Standered deviation" class="Slide (strict)"("Visible"=TRUE) -> ()  [unwired: 2 in, 2 out]
              }
              frame False {
                n161 = call "Simulate Signal29"("Offset"=w523) -> ("DC"=w522:dynamicdata)  [unwired: 13 in, 1 out]
                n162 = property on="Noise Amplitude" class="Slide (strict)"("Visible"=FALSE) -> ()  [unwired: 2 in, 2 out]
                n163 = property on="Trail probability" class="Slide (strict)"("Visible"=FALSE) -> ()  [unwired: 2 in, 2 out]
                n164 = property on="Duty Cycle (%)" class="Knob (strict)"("Visible"=TRUE) -> ()  [unwired: 2 in, 2 out]
                n165 = property on="Standered deviation" class="Slide (strict)"("Visible"=TRUE) -> ()  [unwired: 2 in, 2 out]
              }
            }
          }
          frame 2 {
            n166 = case shown="False" w524 {
              tunnel: w527 -> [w531 w537]
              tunnel: w526 -> [w530 _]
              tunnel: [w529 w536] -> w525
              frame True {
                n167 = call "Simulate Signal15"("Offset"=w531, "Trial probability"=w530) -> ("DC with Binomial Noise"=w529:dynamicdata)  [unwired: 12 in, 1 out]
                n168 = property on="Duty Cycle (%)" class="Knob (strict)"("Visible"=TRUE) -> ()  [unwired: 2 in, 2 out]
                n169 = property on="Noise Amplitude" class="Slide (strict)"("Visible"=FALSE) -> ()  [unwired: 2 in, 2 out]
                n170 = property on="Standered deviation" class="Slide (strict)"("Visible"=FALSE) -> ()  [unwired: 2 in, 2 out]
                n171 = property on="Trail probability" class="Slide (strict)"("Visible"=TRUE) -> ()  [unwired: 2 in, 2 out]
              }
              frame False {
                n172 = call "Simulate Signal30"("Offset"=w537) -> ("DC"=w536:dynamicdata)  [unwired: 13 in, 1 out]
                n173 = property on="Duty Cycle (%)" class="Knob (strict)"("Visible"=TRUE) -> ()  [unwired: 2 in, 2 out]
                n174 = property on="Noise Amplitude" class="Slide (strict)"("Visible"=FALSE) -> ()  [unwired: 2 in, 2 out]
                n175 = property on="Standered deviation" class="Slide (strict)"("Visible"=FALSE) -> ()  [unwired: 2 in, 2 out]
                n176 = property on="Trail probability" class="Slide (strict)"("Visible"=TRUE) -> ()  [unwired: 2 in, 2 out]
              }
            }
          }
        }
      }
    }
    "Sine" <- w36
    "Traingle" <- w35
    "Sawtooth" <- w34
    "Square" <- w33
    "DC" <- w32
    n177 = case shown="True" "Record & Stop Button" {
      tunnel: w7 -> [_ w53]
      tunnel: w6 -> [_ w47]
      tunnel: "File save selector" -> [_ w49]
      frame False {
        n178 = property on="Recorded time" class="DigNum (strict)"("Value"=0.0 ("Recorded time")) -> ()  [unwired: 2 in, 2 out]
      }
      frame True {
        n179 = case shown="\"Radio Selection 1\", Default" w49 {
          tunnel: w53 -> [w54 w55 w56]
          frame "Radio Selection 1", Default {
            n180 = call "Write To Measurement File2"("Signals"=w54) -> ()  [unwired: 16 in, 3 out]
          }
          frame "Radio Selection 2" {
            n181 = call "Write To Measurement File"("Signals"=w55) -> ()  [unwired: 16 in, 3 out]
          }
          frame "Radio Selection 3" {
            n182 = call "Write To Measurement File3"("Signals"=w56) -> ()  [unwired: 16 in, 3 out]
          }
        }
        n183 = Tick Count (ms)() -> (millisecond timer value=w48:u32)
        n184 = Subtract(x=w48, y=w47) -> (x-y=w52:u32)
        n185 = Divide(x=w52, y=u32 1000) -> (x/y=→"Recorded time":dbl)
      }
    }
    n186 = Divide(x=w19, y=5.0) -> (x/y=w16:dbl)
    n187 = Divide(x=w23, y=5.0) -> (x/y=w22:dbl)
    n188 = Divide(x=w16, y=5.0) -> (x/y=w17:dbl)
    n189 = property on="Waveform Graph 2" class="WFGraph (strict)"("YScale.Maximum"=w23, "YScale.Minimum"=w21, "YScale.MinorInc"=w22, "YScale.RngStart"=w21, "YScale.Increment"=w22) -> ()  [unwired: 2 in, 2 out]
    n190 = property on="Waveform Graph 2" class="WFGraph (strict)"("XScale.Maximum"=w19, "XScale.Minimum"=w14, "XScale.MinorInc"=w17, "XScale.RngStart"=w14, "XScale.Increment"=w16) -> ()  [unwired: 2 in, 2 out]
    n191 = case shown="True" "Jpg imgae button" {
      tunnel: "Radio Buttons" -> [_ w66]
      frame False {
      }
      frame True {
        n192 = invoke on="Waveform Graph 2" class="WFGraph (strict)" method="Get Image"() -> ("image data"=w67:T4)  [unwired: 6 in, 5 out]
        n193 = case shown="\"Radio Selection 1\", Default" w66 {
          tunnel: w67 -> [w68 w69 w70]
          frame "Radio Selection 1", Default {
            n194 = call <vilib>:"Write JPEG File.vi"("image data"=w68) -> ()  [unwired: 9 in, 2 out]
          }
          frame "Radio Selection 2" {
            n195 = call <vilib>:"Write PNG File.vi"("image data"=w69) -> ()  [unwired: 9 in, 2 out]
          }
          frame "Radio Selection 3" {
            n196 = call <vilib>:"Write BMP File.vi"("image data"=w70) -> ()  [unwired: 9 in, 2 out]
          }
        }
      }
    }
    n197 = case shown="True" "FFT save button" {
      tunnel: "Radio Buttons" -> [_ w61]
      frame False {
      }
      frame True {
        n198 = invoke on="FFT" class="WFGraph (strict)" method="Get Image"() -> ("image data"=w62:T4)  [unwired: 6 in, 5 out]
        n199 = case shown="\"Radio Selection 3\"" w61 {
          tunnel: w62 -> [w63 w64 w65]
          frame "Radio Selection 1", Default {
            n200 = call <vilib>:"Write JPEG File.vi"("image data"=w63) -> ()  [unwired: 9 in, 2 out]
          }
          frame "Radio Selection 2" {
            n201 = call <vilib>:"Write PNG File.vi"("image data"=w64) -> ()  [unwired: 9 in, 2 out]
          }
          frame "Radio Selection 3" {
            n202 = call <vilib>:"Write BMP File.vi"("image data"=w65) -> ()  [unwired: 9 in, 2 out]
          }
        }
      }
    }
    n203 = call "Tone Measurements"("Signals"=w7) -> ("Frequency"=→"Frequency":dynamicdata, "Amplitude"=→"Peak to Peak Amplitude":dynamicdata)  [unwired: 8 in, 1 out]
    n204 = case shown="True" "Trigger" {
      tunnel: w7 -> [w96 w98]
      tunnel: [w96 w97] -> w30
      frame False {
      }
      frame True {
        n205 = call "Trigger and Gate"("Signals"=w98) -> ("Triggered Signals"=w97:dynamicdata)  [unwired: 7 in, 3 out]
      }
    }
    "Waveform Graph 2" <- w30
    n206 = case shown="\"Waveform\", Default" "Tab Control" {
      frame "Waveform", Default {
        n207 = property on="Jpg imgae button" class="Bool (strict)"("Visible"=TRUE) -> ()  [unwired: 2 in, 2 out]
        n208 = property on="FFT save button" class="Bool (strict)"("Visible"=FALSE) -> ()  [unwired: 2 in, 2 out]
      }
      frame "FFT" {
        n209 = property on="FFT save button" class="Bool (strict)"("Visible"=TRUE) -> ()  [unwired: 2 in, 2 out]
        n210 = property on="Jpg imgae button" class="Bool (strict)"("Visible"=FALSE) -> ()  [unwired: 2 in, 2 out]
      }
    }
    n211 = xnode "Spectral Measurements"("Signals"=w7) -> ("FFT - (Peak)"=→"FFT":dynamicdata)  [unwired: 1 in, 2 out]
    n212 = Not(x="stop") -> (.not. x?=→".not. x?":bool)
  }
